vi "Run_Tests_CLI.vi"(11 "Command Line Arguments":string[](array[string])) -> (2 "Output":string, 3 "Exit Code":i32)   [LabVIEW 2025]
uses:
  <vilib>/addons/_JKI Toolkits/Caraya/classes/Test Suite/Test Suite.lvclass
  <vilib>/addons/_JKI Toolkits/Caraya/classes/Test Suite/Define Test Suite (Default).vi
  MCP Server tests.lvlib
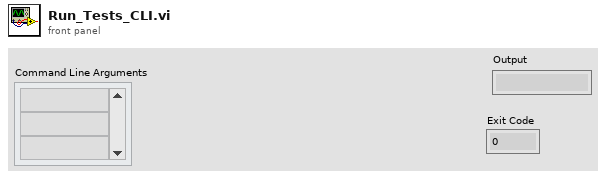
[diagram p1: front panel]
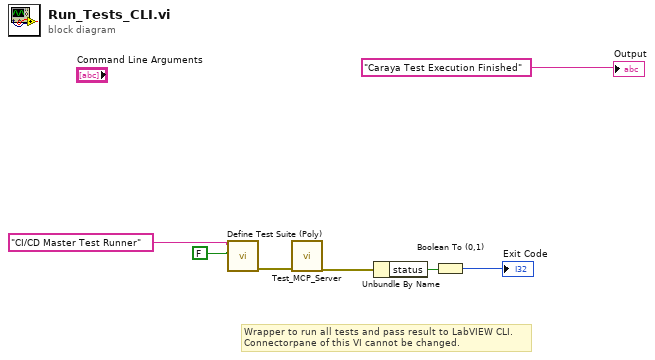
[diagram p0: block diagram]
diagram:
  # "Wrapper to run all tests and pass result to LabVIEW CLI.\nConnectorpane of this VI cannot be changed."
  n1 = call-poly <vilib>:"Define Test Suite (Poly).vi"("Interactive"=FALSE, "Label (VI Title)"="CI/CD Master Test Runner") -> ("error out"=w6:errorcluster)  [unwired: 7 in, 2 out]
  n2 = call "Test_MCP_Server.vi"("error in (no error)"=w6) -> ("error out"=w4:errorcluster)  [unwired: 10 in]
  n3 = Unbundle By Name(w4) -> ("status"=w3:bool)
  n4 = Boolean To (0,1)(Boolean=w3) -> (0, 1=→"Exit Code":i16)
  "Output" <- "Caraya Test Execution Finished" ("Output")
